vi "SigProc_method appendYData.vi"(0 "error in (no error)":errorcluster) -> (2 "error out":errorcluster)   [LabVIEW 2018, in "Sig2MS.lvclass"]
uses:
  Sig2MS.lvclass
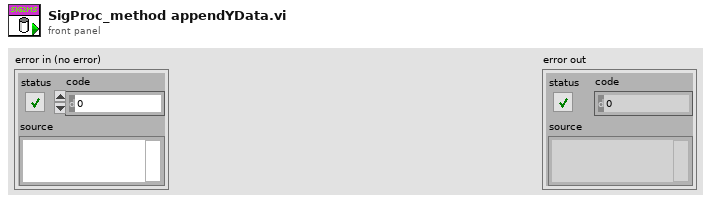
[diagram p1: front panel]
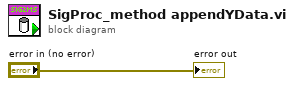
[diagram p0: block diagram]
diagram:
  "error out" <- "error in (no error)"
